vi "ni579x Host Align 2.vi"(0 "sync.resources":T1, 1 "sync.meas.Reference Clock":refnum<k21>, 2 "sync.meas.FPGA I/O":refnum<k21>) -> (4 "sync.resources":T1)   [LabVIEW 2013, in "ni579x Synchronization v1 FPGA.lvlib"]
doc: "Align the targets participating in synchronization. This must occur before a signal can be synchronized.\n\nThere are two flavors of alignment to chose from -- Host Align and FPGA Align. The two flavors produce the same quality of synchronization, but differ in requirements and versatility of operation.\n\nWhen using <B>ni579x FPGA Align</B>, the Single Cycle Timed Loop (SCTL) rate (that this VI is in) must be an integer multiple of the <B>sync.cptr.Reference Clock</B> rate, and the SCTL clock must have a fixed phase relationship to the reference clock. Each target performs its alignment independently, so FPGA Align does not require a FPGA I/O line. It's also possible to use FPGA Align without host interaction. FPGA Align has 100% repeatability if-and-only-if the target-to-target phase relationship is low and does not change.\n\nWhen using <B>ni579x Host Align</B>, the SCTL rate may be arbitrary (yet still must have a fixed phase relationship to the other targets). The CPTR period may also be arbitrary. This alignment process is coordinated by the host, and requires an FPGA I/O line for orchestration. Host Align has 100% repeatability; if the hardware configuration remains constant, so will the level of synchronization.\n\n<B>Input Parameters</B>\n\n<B>sync.resources</B> identifies the Synchronization instance. 'sync.resources' is obtained from the ni579x Create VI of this library.\n\n<B>sync.meas.Reference Clock</B> is used by the measurement logic as the \"start\" signal. This is commonly PXI_Clk10.\n\n<B>sync.meas.FPGA I/O</B> is the FPGA I/O line that will be used to orchestrate starting the measurements. This is commonly a PXI Trig line.\n\nNote: For large NI chassis, make sure the PXI Trig line is routed to all bus segments that have targets participating in synchronization.\n\n<B>Output Parameters</B>\n\n<B>sync.resources</B> is the same instance that was passed in for 'sync.resources'."
uses:
  <instrlib>/ni579x/Synchronization/v1/FPGA/ni579x Synchronization v1 FPGA.lvlib
  <instrlib>/ni579x/Synchronization/v1/FPGA/Implementation/Resources.ctl
  <vilib>/rvi/eio/common/nirviEmuTemplateMethod_errors.vi
  <vilib>/eio/EIONode/EIONode.xnode
  <instrlib>/_niInstr/Basic Elements/v1/FPGA/niInstr Basic Elements v1 FPGA.lvlib
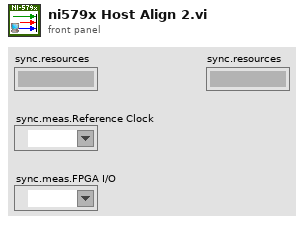
[diagram p1: front panel]
types:
  T1 = typedef "ni579x Synchronization v1 FPGA.lvlib/Resources.ctl" = cluster{"master":refnum<k21>, "meas.enable":refnum<k21>, "meas.ready":refnum<k21>, "meas.arm":refnum<k21>, "meas.valid":refnum<k21>, "meas.value":refnum<k21>, "meas.oversample clock":refnum<k21>, "meas.oversample factor":refnum<k21>, "cptr":refnum<k21>, "cptr.adjust":refnum<k21>, "cptr.period":refnum<k21>}
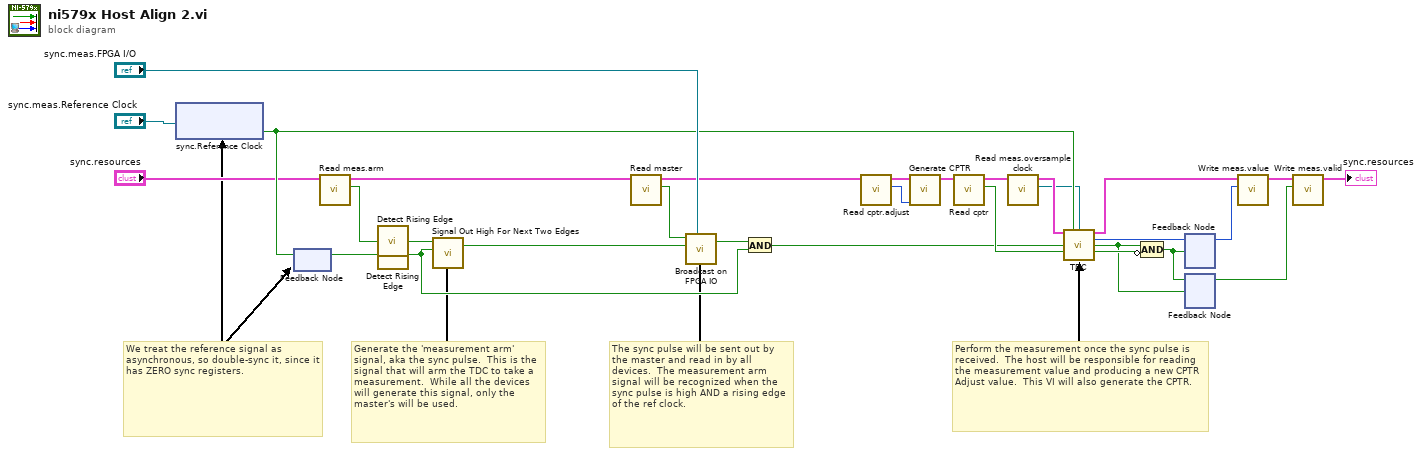
[diagram p0: block diagram]
diagram:
  # "We treat the reference signal as asynchronous, so double-sync it, since it has ZERO sync registers."
  # "Perform the measurement once the sync pulse is received.  The host will be responsible for reading the measurement value and producing a new CPTR Adjust value.  This VI will also generate the CPTR."
  # "The sync pulse will be sent out by the master and read in by all devices.  The measurement arm signal will be recognized when the sync pulse is high AND a rising edge of the ref clock."
  # "Generate the 'measurement arm' signal, aka the sync pulse.  This is the signal that will arm the TDC to take a measurement.  While all the devices will generate this signal, only the master's will be used."
  n1 = xnode ("sync.Reference Clock")("FPGA I/O In"="sync.meas.Reference Clock") -> ("I/O Item"=w20:bool)  [unwired: 1 out]
  n2 = feedback #1() -> (w27:bool)  [unwired: 1 in]
  n3 = feedback-in #1(w20) -> ()
  n4 = call <instrlib>:"Read meas.arm.vi"("sync.resources"="sync.resources") -> ("meas.arm"=w23:bool, "sync.resources"=w14:T1)  [unwired: 9 in]
  n5 = call <instrlib>:"Detect Rising Edge.vi"("signal"=w23) -> ("edge detected"=w28:bool)  [unwired: 14 in]
  n6 = call <instrlib>:"Detect Rising Edge.vi"("signal"=w27) -> ("edge detected"=w30:bool)  [unwired: 14 in]
  n7 = call <instrlib>:"Signal Out High For Next Two Edges.vi"("edge"=w30, "signal"=w28) -> ("signal for distribution"=w26:bool)  [unwired: 3 in]
  n8 = call <instrlib>:"Read master.vi"("sync.resources"=w14) -> ("master"=w22:bool, "sync.resources"=w9:T1)  [unwired: 9 in]
  n9 = call <instrlib>:"Broadcast on FPGA IO.vi"("FPGA I/O"="sync.meas.FPGA I/O", "signal in"=w26, "master"=w22) -> ("signal out"=w25:bool)  [unwired: 4 in]
  n10 = And(x=w25, y=w30) -> (x .and. y?=w15:bool)
  n11 = call <instrlib>:"Read cptr.adjust.vi"("sync.resources"=w9) -> ("cptr.adjust"=w8:u16, "sync.resources"=w10:T1)  [unwired: 9 in]
  n12 = call <instrlib>:"Generate CPTR.vi"("sync.cptr.adjust"=w8, "sync.resources"=w10) -> ("sync.resources"=w7:T1)  [unwired: 9 in]
  n13 = call <instrlib>:"Read cptr.vi"("sync.resources"=w7) -> ("cptr"=w21:bool, "sync.resources"=w4:T1)  [unwired: 9 in]
  n14 = call <instrlib>:"Read meas.oversample clock.vi"("sync.resources"=w4) -> ("meas.oversample clock"=w1:refnum<k21>, "sync.resources"=w2:T1)  [unwired: 9 in]
  n15 = call <instrlib>:"TDC.vi"("sync.resources"=w2, "sync.Reference Clock"=w20, "sync.meas.oversample clock"=w1, "sync.meas.arm"=w15, "sync.cptr"=w21) -> ("sync.resources"=w3:T1, "count out"=w18:u16, "count valid"=w11:bool, "rollover error"=w12:bool)  [unwired: 6 in, 1 out]
  n16 = Compound Arithmetic op=AND(w11, invert w12) -> (w19:bool)
  n17 = feedback #2() -> (w17:u16)  [unwired: 1 in]
  n18 = feedback-in #2(w18, w19) -> ()
  n19 = feedback #3() -> (w16:bool)  [unwired: 1 in]
  n20 = feedback-in #3(w19, w11) -> ()
  n21 = call <instrlib>:"Write meas.value.vi"("meas.value"=w17, "sync.resources"=w3) -> ("sync.resources"=w13:T1)  [unwired: 9 in]
  n22 = call <instrlib>:"Write meas.valid.vi"("meas.valid"=w16, "sync.resources"=w13) -> ("sync.resources"=→"sync.resources":T1)  [unwired: 9 in]
